vi "Get part type.vi"(11 "Enum":T1) -> (3 "Parttype":string)   [LabVIEW 2014]
uses:
  typedefs/parttype.ctl
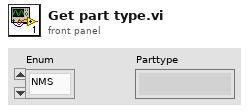
[diagram p1: front panel]
types:
  T1 = typedef "parttype.ctl" = enum16{"NMS", "B-SUV"}
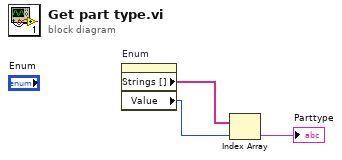
[diagram p0: block diagram]
diagram:
  n1 = property on="Enum" class="Enum (strict)"() -> ("Strings []"=w3:string[], "Value"=w2:T1)  [unwired: 2 in, 2 out]
  n2 = Index Array(array=w3, index=w2) -> (element=→"Parttype":string)
